vi "Constructor.vi"(8 "error in (no error)":errorcluster, 11 "Singleton.lvclass In":refnum<class "Singleton.lvclass">) -> (0 "error out":errorcluster, 3 "SingletonDVR Out":refnum<data-value>)   [LabVIEW 2014, in "Singleton.lvclass"]
uses:
  Singleton.lvclass
  Singleton.lvclass/Singleton.ctl
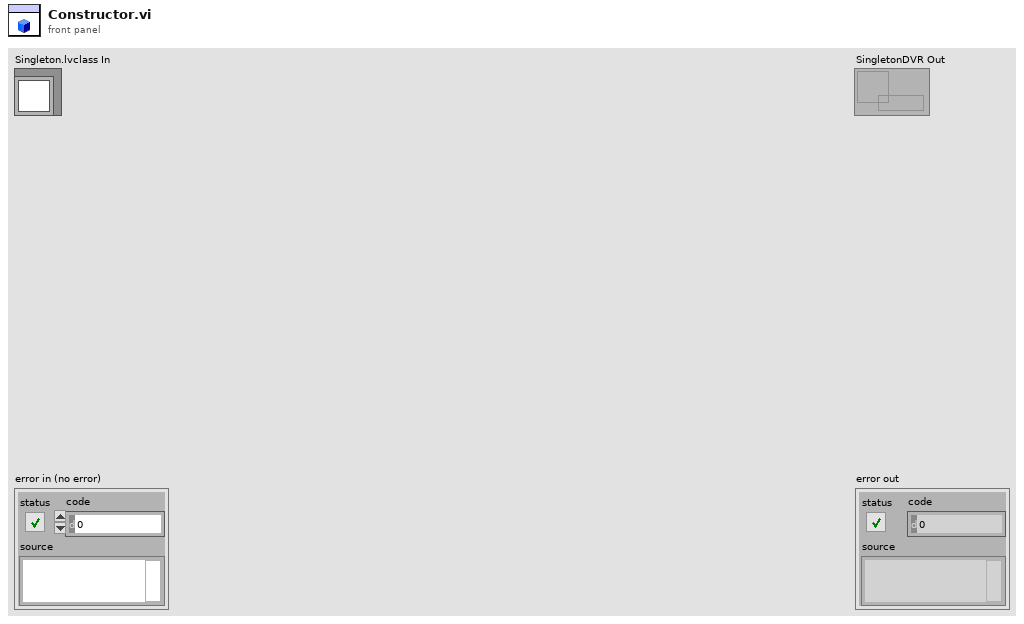
[diagram p1: front panel]
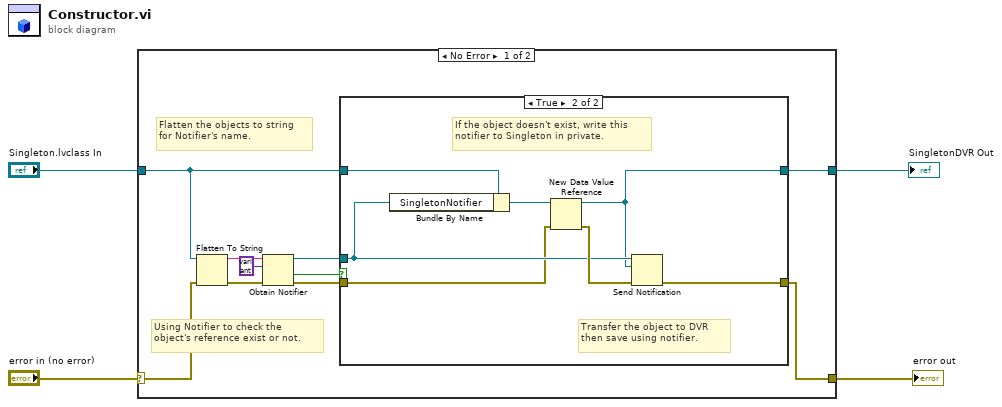
[diagram p0: block diagram]
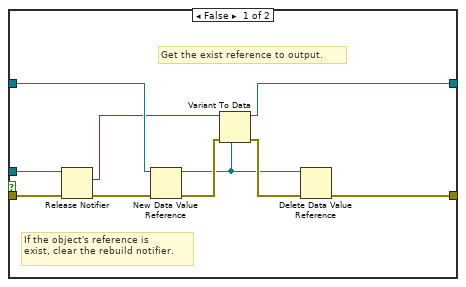
[diagram p2: hidden frame]
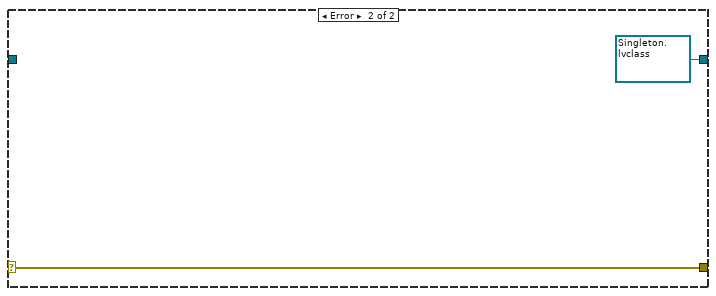
[diagram p3: hidden frame]
diagram:
  n1 = case shown="No Error" "error in (no error)" {
    selector: "error in (no error)" -> [w14 w33]
    tunnel: [w5 w33] -> w3
    tunnel: "Singleton.lvclass In" -> [w8 _]
    tunnel: [w6 refnum<data-value> refnum ("data value reference")] -> w1
    frame No Error {
      # "Using Notifier to check the\nobject's reference exist or not."
      # "Flatten the objects to string\nfor Notifier's name."
      n2 = Flatten To String(anything=w8, error in (no error)=w14) -> (data string=w12:string, error out=w13:errorcluster)  [unwired: 2 in, 1 out]
      n3 = Obtain Notifier(name (unnamed)=w12, notification data type=variant ("element data type"), error in (no error)=w13) -> (notifier out=w9:refnum<notifier>, created new?=w10:bool, error out=w7:errorcluster)  [unwired: 1 in]
      n4 = case shown="True" w10 {
        tunnel: w9 -> [w23 w28]
        tunnel: w8 -> [w21 w31]
        tunnel: w7 -> [w24 w25]
        tunnel: [w19 w27] -> w6
        tunnel: [w15 w26] -> w5
        frame False {
          # "Get the exist reference to output."
          # "If the object's reference is\nexist, clear the rebuild notifier."
          n5 = Release Notifier(notifier=w23, error in (no error)=w24) -> (last notification=w20:variant, error out=w22:errorcluster)  [unwired: 1 in, 1 out]
          n6 = New Data Value Reference(data value=w21, error in=w22) -> (data value reference=w16:refnum<data-value>, error out=w18:errorcluster)
          n7 = Variant To Data(error in=w18, type=w16, Variant=w20) -> (data=w19:refnum<data-value>, error out=w17:errorcluster)
          n8 = Delete Data Value Reference(data value reference=w16, error in=w17) -> (error out=w15:errorcluster)  [unwired: 1 out]
        }
        frame True {
          # "Transfer the object to DVR\nthen save using notifier."
          # "If the object doesn't exist, write this\nnotifier to Singleton in private."
          n9 = Bundle By Name(cluster=w31, "SingletonNotifier"=w28) -> (w30:refnum<class "Singleton.lvclass">)
          n10 = New Data Value Reference(data value=w30, error in=w25) -> (data value reference=w27:refnum<data-value>, error out=w29:errorcluster)
          n11 = Send Notification(notification=w27, notifier=w28, error in (no error)=w29) -> (error out=w26:errorcluster)  [unwired: 1 out]
        }
      }
    }
    frame Error {
    }
  }
  "error out" <- w3
  "SingletonDVR Out" <- w1
